vi "Station Position Status.vi"(6 "error in (no error)":errorcluster, 7 "Wash Steps Selected-Update Display Message":T1, 8 "Car Wash References":T2) -> (0 "error out":errorcluster, 1 "Message Out":T1)   [LabVIEW 2020]
doc: "This VI checks if the car position is correct or incorrect for the current wash step and pdates the Display Message."
uses:
  Controls/Car Wash References.ctl
  Controls/Wash Steps Selected-Update Display Message.ctl
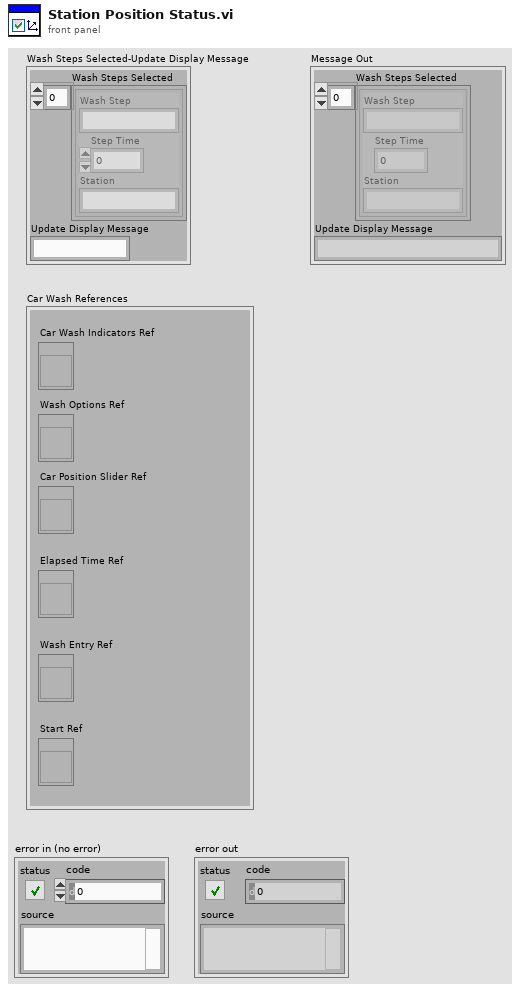
[diagram p1: front panel]
types:
  T1 = typedef "Wash Steps Selected-Update Display Message.ctl" = cluster{"Wash Steps Selected":cluster{"Wash Step":string, "Step Time":i32, "Station":string}[], "Update Display Message":string}
  T2 = typedef "Car Wash References.ctl" = cluster{"Car Wash Indicators Ref":refnum<vi>, "Wash Options Ref":refnum<vi>, "Car Position Slider Ref":refnum<vi>, "Elapsed Time Ref":refnum<vi>, "Wash Entry Ref":refnum<vi>, "Start Ref":refnum<vi>}
  T3 = cluster{"Wash Step":string, "Step Time":i32, "Station":string}[]
  T4 = cluster{"Wash Step":string, "Step Time":i32, "Station":string}
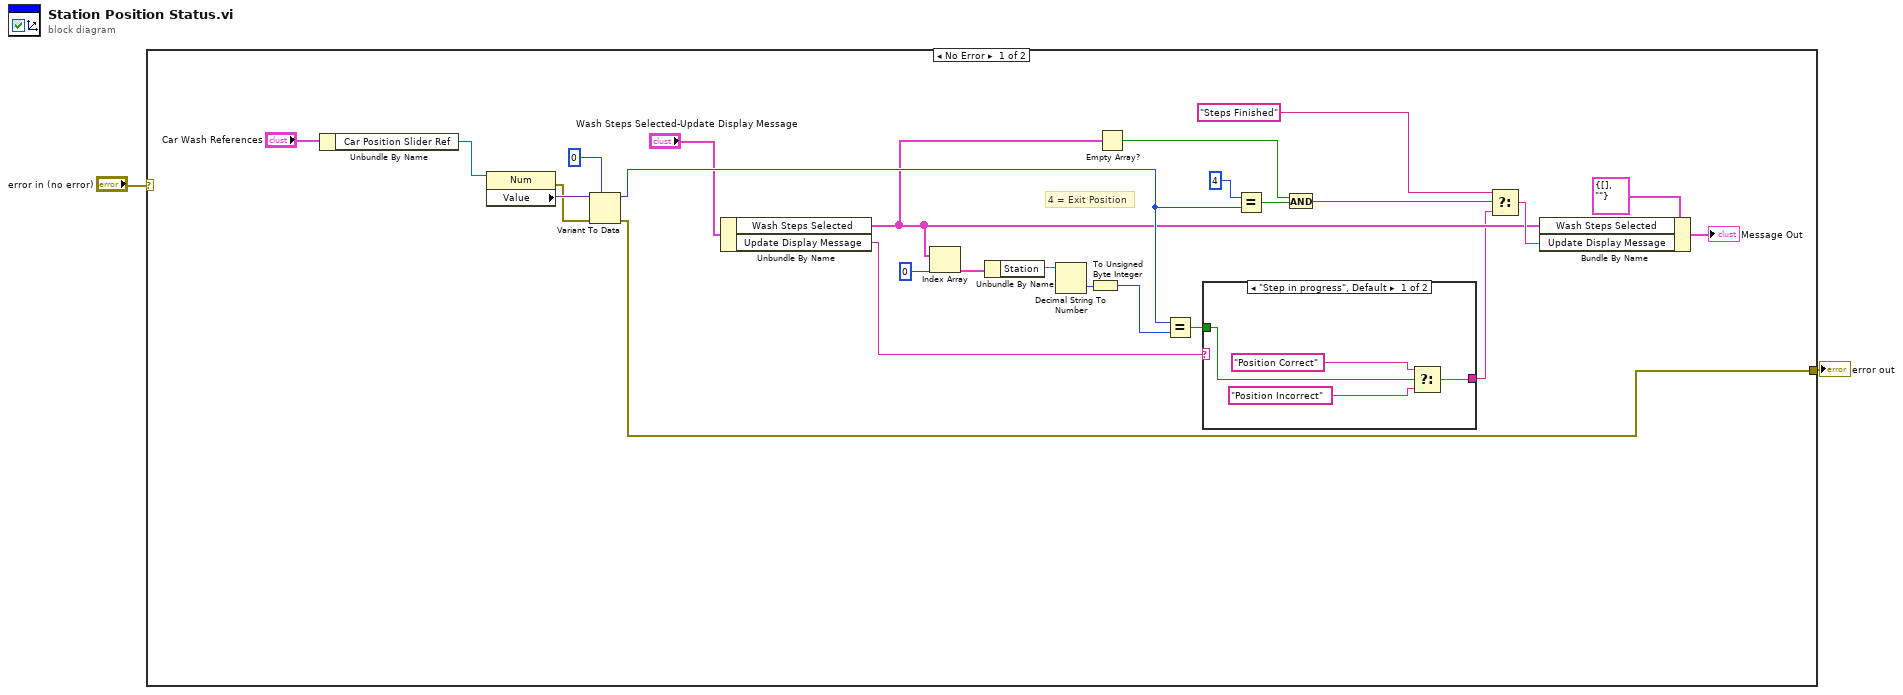
[diagram p0: block diagram]
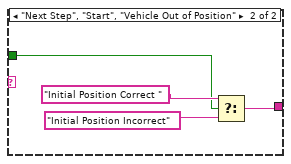
[diagram p2: hidden frame]
diagram:
  n1 = case shown="No Error" "error in (no error)" {
    selector: "error in (no error)" -> [_ w36]
    tunnel: [w7 w36] -> w2
    frame No Error {
      # "4 = Exit Position"
      n2 = Unbundle By Name("Car Wash References") -> ("Car Position Slider Ref"=w26:refnum<vi>)
      n3 = property class="Num"(reference=w26) -> (error out=w23:errorcluster, "Value"=w25:variant)  [unwired: 1 in, 1 out]
      n4 = Variant To Data(error in=w23, type=u8 0, Variant=w25) -> (data=w14:u8, error out=w7:errorcluster)
      n5 = Unbundle By Name("Wash Steps Selected-Update Display Message") -> ("Wash Steps Selected"=w4:T3, "Update Display Message"=w6:string)
      n6 = Index Array(array=w4, index=0) -> (element=w21:T4)
      n7 = Unbundle By Name(w21) -> ("Station"=w20:string)
      n8 = Decimal String To Number(string=w20) -> (number=w17:i32)  [unwired: 2 in, 1 out]
      n9 = To Unsigned Byte Integer(number=w17) -> (unsigned 8bit integer=w10:u8)
      n10 = Empty Array?(array=w4) -> (empty?=w16:bool)
      n11 = Equal?(x=w14, y=w10) -> (x = y?=w5:bool)
      n12 = case shown="\"Step in progress\", Default" w6 {
        tunnel: w5 -> [w29 w32]
        tunnel: [w28 w33] -> w3
        frame "Step in progress", Default {
          n13 = Select(t="Position Correct", s=w29, f="Position Incorrect") -> (s? t:f=w28:string)
        }
        frame "Next Step", "Start", "Vehicle Out of Position" {
          n14 = Select(t="Initial Position Correct ", s=w32, f="Initial Position Incorrect") -> (s? t:f=w33:string)
        }
      }
      n15 = Equal?(x=u8 4 ("index"), y=w14) -> (x = y?=w13:bool)
      n16 = And(x=w16, y=w13) -> (x .and. y?=w12:bool)
      n17 = Select(t="Steps Finished", s=w12, f=w3) -> (s? t:f=w9:string)
      n18 = Bundle By Name(cluster=T1 {"Wash Steps Selected"=[], "Update Display Message"=""}, "Wash Steps Selected"=w4, "Update Display Message"=w9) -> (→"Message Out":T1)
    }
    frame Error {
    }
  }
  "error out" <- w2
